vi "linspace.vi"(9 "Nvalues":i32, 10 "Stop":dbl, 11 "Start":dbl) -> (3 "Array":dbl[](array[numeric]))   [LabVIEW 2015]
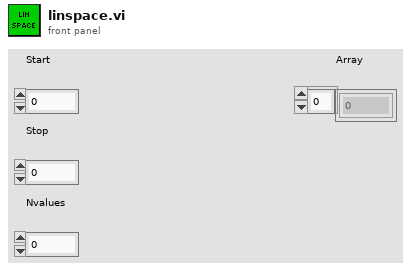
[diagram p1: front panel]
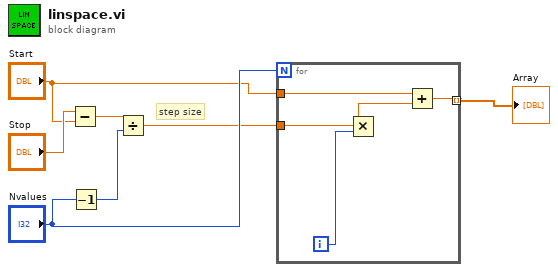
[diagram p0: block diagram]
diagram:
  # "step size"
  n1 = Subtract(x="Stop", y="Start") -> (x-y=w6:dbl)
  n2 = Decrement(x="Nvalues") -> (x-1=w5:i32)
  n3 = Divide(x=w6, y=w5) -> (x/y=w2:dbl)
  n4 = for {
    N: "Nvalues" -> [_]
    tunnel: "Start" -> [w10]
    tunnel: w2 -> [w12]
    tunnel: [w8] -> w1 mode=indexing
    i -> [w11]
    n5 = Multiply(x=w12, y=w11) -> (x*y=w9:dbl)
    n6 = Add(x=w10, y=w9) -> (x+y=w8:dbl)
  }
  "Array" <- w1
